vi "SUB-ROM Data convert to table.vi"(4 "ROM Table Ref":refnum<vi>, 5 "ROM Data Ref":refnum<vi>) -> (1 "ROM Table":string[][](table)=[["Device ID", "-", "-"], ["Main Chip", "-", "-"], ["YEAR", "-", "-"], ["Month", "-", "-"], ["Day", "-", "-"], ["Device Type", "-", "-"], ["Manufacturer ID", "-", "-"], ["Cal_Acc. X", "-", "-"], ["Cal_Acc. Y", "-", "-"], ["Cal_Acc. Z", "-", "-"], ["Cal_Gy. X", "-", "-"], ["Cal_Gy. Y", "-", "-"], ["Cal_Gy. Z", "-", "-"], ["Cal_Vol H", "-", "-"], ["Cal_Vol L", "-", "-"], ["Cal_CDC Off 1", "-", "-"], ["Cal_CDC Off 2", "-", "-"], ["Cal_CDC Off 3", "-", "-"], ["Cal_CDC Off 4", "-", "-"], ["Cal_CDC Off 5", "-", "-"], ["Cal_CDC Off 6", "-", "-"], ["Cal_CDC Gain A", "-", "-"], ["Cal_CDC Gain B", "-", "-"]], 2 "ROM Data":T1(array[cluster])=[{"RxOK"=TRUE, "ROM Data"=[255, 255, 255, 255, 255, 255, 255, 255, 255, 255, 255, 255, 255, 255, 255, 255, 2], "Index"=0}, {"RxOK"=TRUE, "ROM Data"=[255, 255, 255, 255, 255, 255, 255, 255, 255, 255, 255, 255, 255, 255, 255, 255, 5], "Index"=1}, {"RxOK"=TRUE, "ROM Data"=[255, 255, 255, 255, 255, 255, 255, 255, 255, 255, 255, 255, 255, 255, 255, 255, 8], "Index"=2}] {"Index" format="%02x"; "ROM Data" format="%02x"})   [LabVIEW 2015]
panel:
  out "Last Index":i32=2
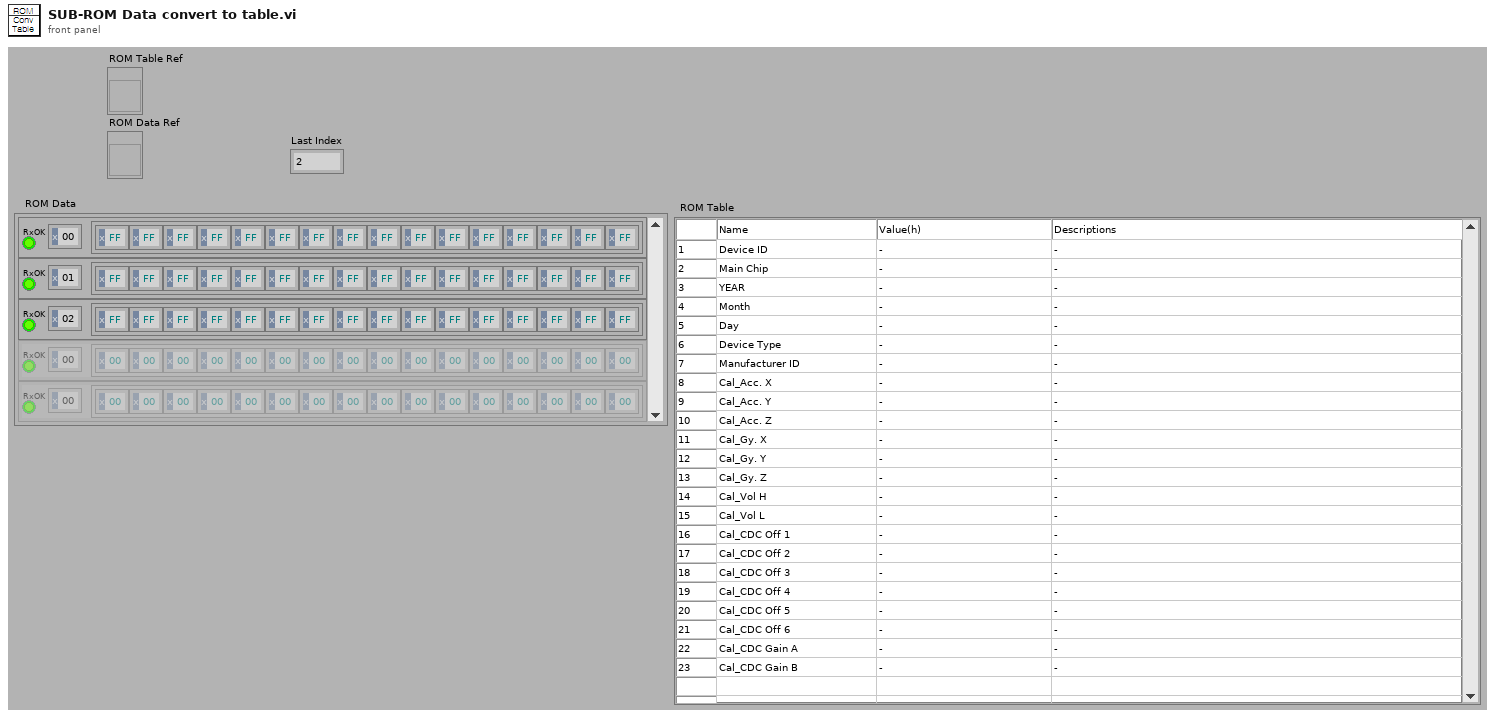
[diagram p1: front panel]
types:
  T1 = cluster{"RxOK":bool, "ROM Data":u8[], "Index":u8}[]
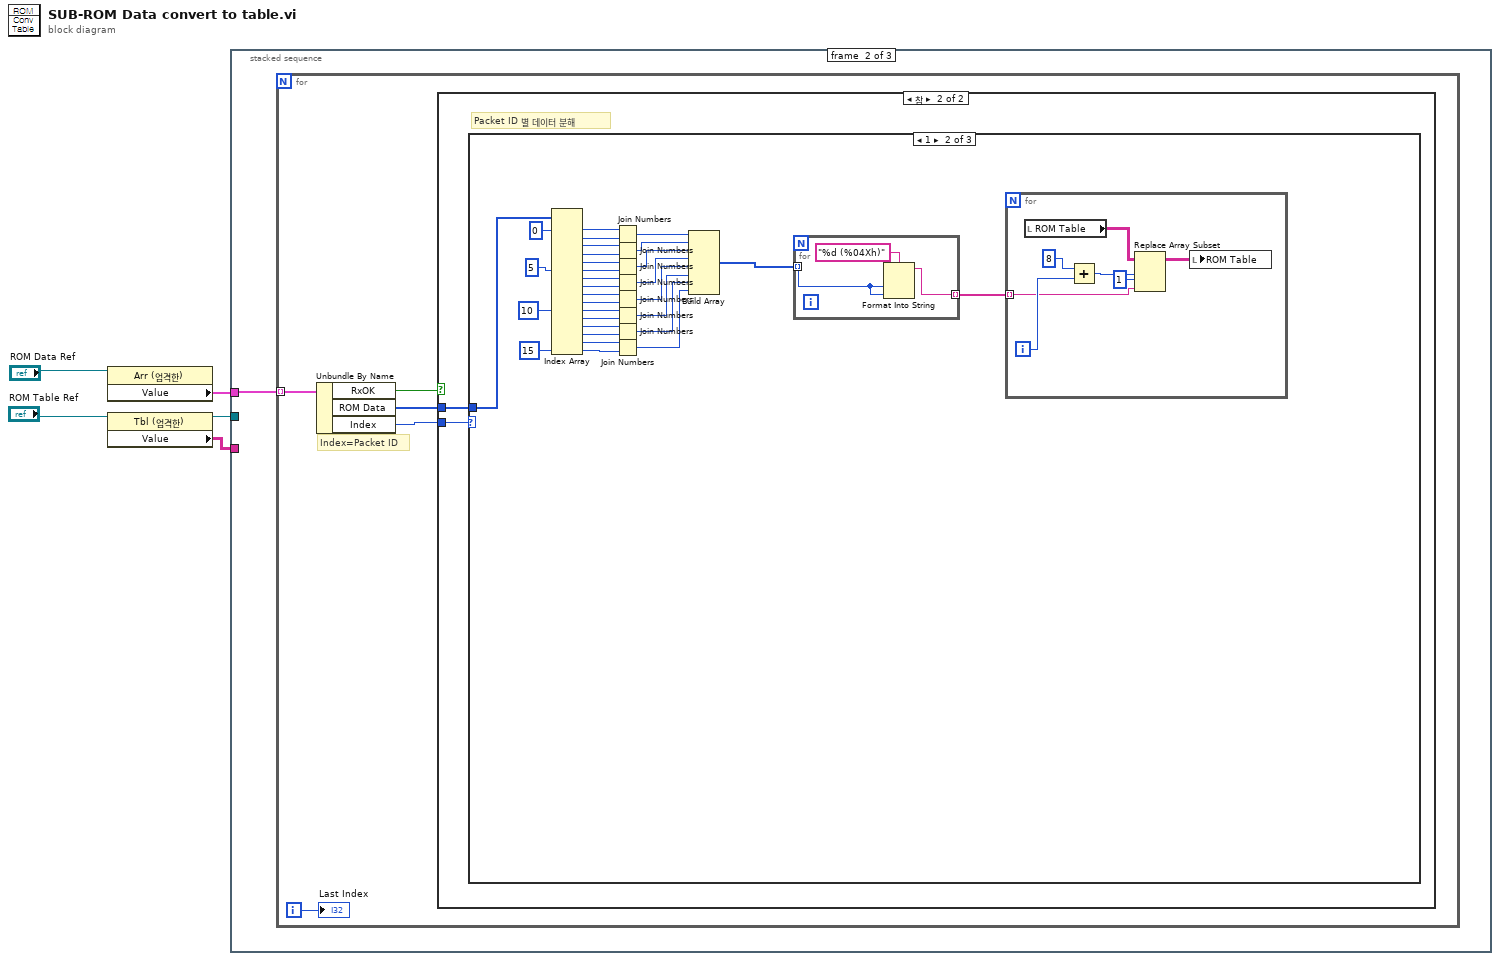
[diagram p0: block diagram]
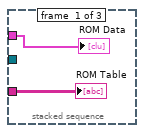
[diagram p2: hidden frame]
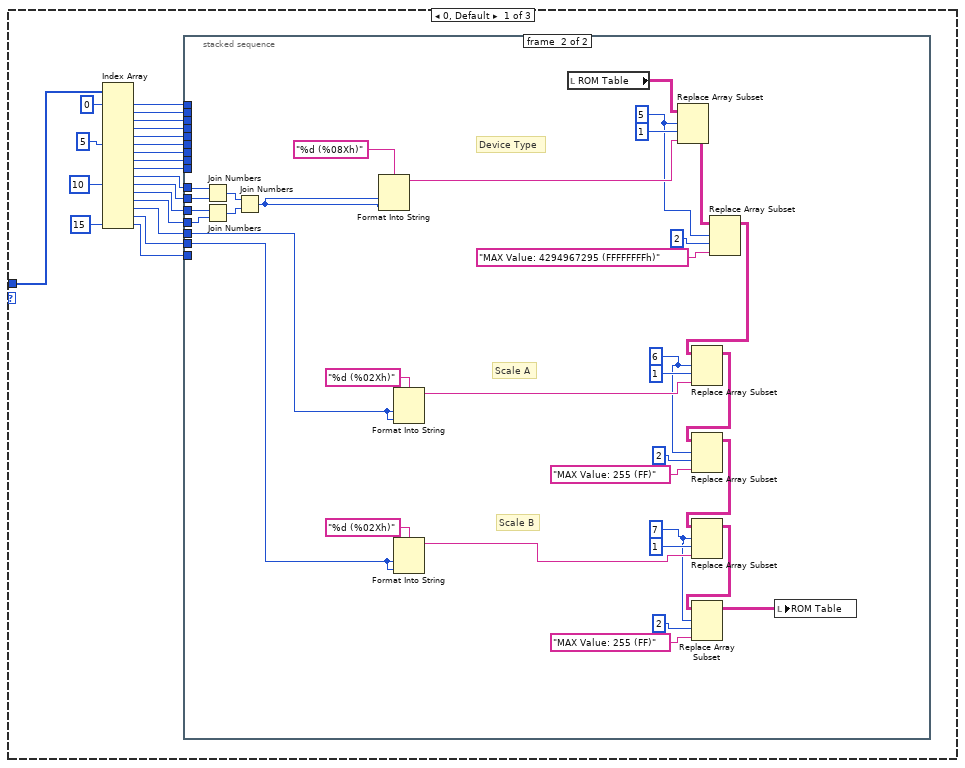
[diagram p4: hidden frame]
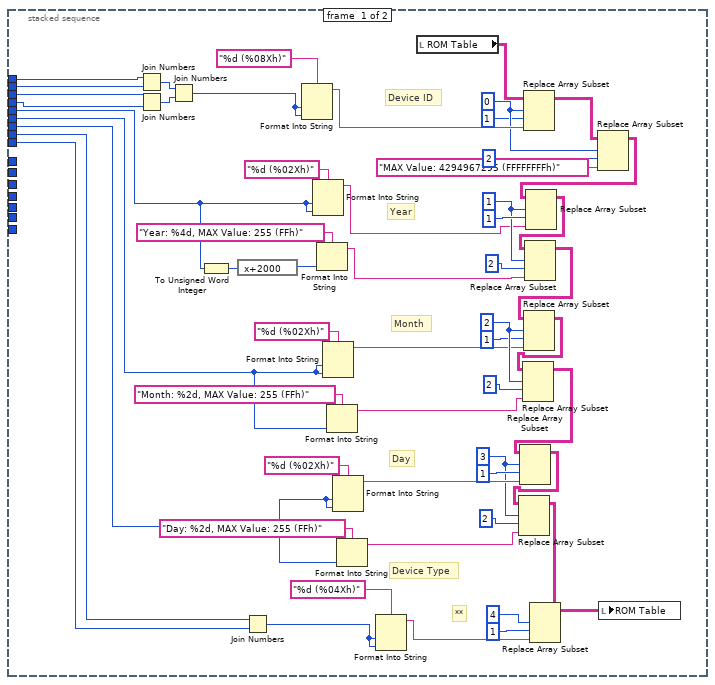
[diagram p5: hidden frame]
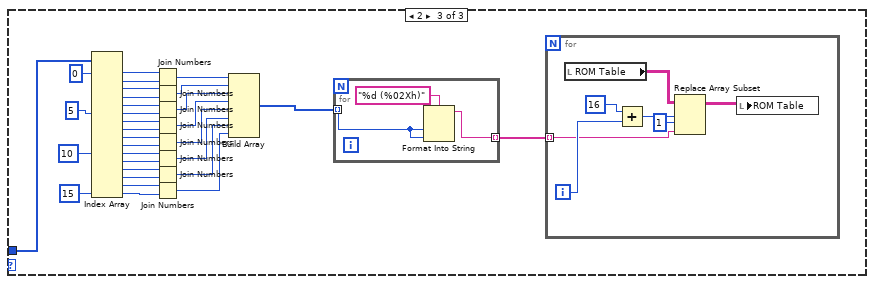
[diagram p6: hidden frame]
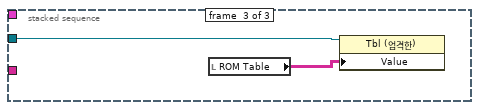
[diagram p7: hidden frame]
diagram:
  n1 = property class="Arr (엄격한)"(reference="ROM Data Ref") -> ("Value"=w3:T1)  [unwired: 1 in, 2 out]
  n2 = property class="Tbl (엄격한)"(reference="ROM Table Ref") -> (reference out=w1:refnum<vi>, "Value"=w2:string[][])  [unwired: 1 in, 1 out]
  n3 = stacked-sequence {
    tunnel: w3 -> [w7 w8 _]
    tunnel: w2 -> [w6 _ _]
    tunnel: w1 -> [_ _ w210]
    frame #0 {
      "ROM Data" <- w7
      "ROM Table" <- w6
    }
    frame #1 {
      n4 = for {
        tunnel: w8 -> [w13] mode=indexing
        i -> [w9]
        # "Index=Packet ID"
        n5 = Unbundle By Name(w13) -> ("RxOK"=w11:bool, "ROM Data"=w10:u8[], "Index"=w12:u8)
        n6 = case shown="참" w11 {
          tunnel: w12 -> [_ w15]
          tunnel: w10 -> [_ w14]
          frame False {
          }
          frame True {
            # "Packet ID 별 데이터 분해"
            n7 = case shown="1" w15 {
              tunnel: w14 -> [w32 w153 w194]
              frame 0, Default {
                n8 = Index Array(array=w32, index #1=0 ("인덱스"), index #6=5 ("인덱스"), index #11=10 ("인덱스"), index #16=15 ("인덱스")) -> (element #1=w31:u8, element #2=w30:u8, element #3=w29:u8, element #4=w28:u8, element #5=w27:u8, element #6=w26:u8, element #7=w25:u8, element #8=w24:u8, element #9=w23:u8, element #10=w22:u8, element #11=w21:u8, element #12=w20:u8, element #13=w19:u8, element #14=w18:u8, element #15=w17:u8, element #16=w16:u8)  [unwired: 12 in]
                n9 = stacked-sequence {
                  tunnel: w31 -> [w87 _]
                  tunnel: w30 -> [w86 _]
                  tunnel: w29 -> [w85 _]
                  tunnel: w28 -> [w84 _]
                  tunnel: w27 -> [w78 _]
                  tunnel: w26 -> [w64 _]
                  tunnel: w25 -> [w52 _]
                  tunnel: w24 -> [w46 _]
                  tunnel: w23 -> [w45 _]
                  tunnel: w22 -> [_ w124]
                  tunnel: w21 -> [_ w123]
                  tunnel: w20 -> [_ w122]
                  tunnel: w19 -> [_ w121]
                  tunnel: w18 -> [_ w113]
                  tunnel: w17 -> [_ w110]
                  tunnel: w16 -> [_ _]
                  frame #0 {
                    w56 = 3 ("인덱스 (행)")
                    w69 = 2 ("인덱스 (행)")
                    w75 = 1 ("인덱스 (행)")
                    w42 = 0 ("인덱스 (행)")
                    # "Device Type"
                    # "**"
                    # "Day"
                    # "Month"
                    # "Year"
                    # "Device ID"
                    n10 = Join Numbers(hi=w87, lo=w86) -> ((hi.lo)=w88:u16)
                    n11 = Join Numbers(hi=w85, lo=w84) -> ((hi.lo)=w89:u16)
                    n12 = Join Numbers(hi=w88, lo=w89) -> ((hi.lo)=w91:u32)
                    n13 = To Unsigned Word Integer(number=w78) -> (unsigned 16bit integer=w79:u16)
                    n14 = expression code="x+2000"(w79) -> (w80:u16)
                    n15 = Join Numbers(hi=w46, lo=w45) -> ((hi.lo)=w50:u16)
                    n16 = Format Into String(format string="%d (%08Xh)" ("포맷 문자열"), w91, w91) -> (resulting string=w83:string)  [unwired: 2 in, 1 out]
                    n17 = Format Into String(format string="%d (%02Xh)" ("포맷 문자열"), w78, w78) -> (resulting string=w73:string)  [unwired: 2 in, 1 out]
                    n18 = Format Into String(format string="Year: %4d, MAX Value: 255 (FFh)" ("포맷 문자열"), w80) -> (resulting string=w72:string)  [unwired: 2 in, 1 out]
                    n19 = Format Into String(format string="%d (%02Xh)" ("포맷 문자열"), w64, w64) -> (resulting string=w67:string)  [unwired: 2 in, 1 out]
                    n20 = Format Into String(format string="Month: %2d, MAX Value: 255 (FFh)" ("포맷 문자열"), w64) -> (resulting string=w71:string)  [unwired: 2 in, 1 out]
                    n21 = Format Into String(format string="%d (%02Xh)" ("포맷 문자열"), w52, w52) -> (resulting string=w59:string)  [unwired: 2 in, 1 out]
                    n22 = Format Into String(format string="Day: %2d, MAX Value: 255 (FFh)" ("포맷 문자열"), w52) -> (resulting string=w54:string)  [unwired: 2 in, 1 out]
                    n23 = Format Into String(format string="%d (%04Xh)" ("포맷 문자열"), w50, w50) -> (resulting string=w48:string)  [unwired: 2 in, 1 out]
                    n24 = local read "ROM Table"() -> (w92:string[][])
                    n25 = Replace Array Subset(array=w92, new element=w83, index (row)=w42, index (col)=1 ("비활성화된 인덱스 (열)")) -> (w44:string[][])
                    n26 = Replace Array Subset(array=w44, new element="MAX Value: 4294967295 (FFFFFFFFh)" ("새 원소/부분배열"), index (row)=w42, index (col)=2 ("비활성화된 인덱스 (열)")) -> (w43:string[][])
                    n27 = Replace Array Subset(array=w43, new element=w73, index (row)=w75, index (col)=1 ("인덱스 (행)")) -> (w74:string[][])
                    n28 = Replace Array Subset(array=w74, new element=w72, index (row)=w75, index (col)=2 ("인덱스 (행)")) -> (w63:string[][])
                    n29 = Replace Array Subset(array=w63, new element=w67, index (row)=w69, index (col)=1 ("인덱스 (행)")) -> (w62:string[][])
                    n30 = Replace Array Subset(array=w62, new element=w71, index (row)=w69, index (col)=2 ("인덱스 (행)")) -> (w53:string[][])
                    n31 = Replace Array Subset(array=w53, new element=w59, index (row)=w56, index (col)=1 ("인덱스 (행)")) -> (w57:string[][])
                    n32 = Replace Array Subset(array=w57, new element=w54, index (row)=w56, index (col)=2 ("인덱스 (행)")) -> (w47:string[][])
                    n33 = Replace Array Subset(array=w47, new element=w48, index (row)=4 ("인덱스 (행)"), index (col)=1 ("인덱스 (행)")) -> (w37:string[][])
                    n34 = local write "ROM Table"(w37) -> ()
                  }
                  frame #1 {
                    w99 = 7 ("인덱스 (행)")
                    w98 = 6 ("인덱스 (행)")
                    w93 = 5 ("인덱스 (행)")
                    # "Scale B"
                    # "Scale A"
                    # "Device Type"
                    n35 = Join Numbers(hi=w124, lo=w123) -> ((hi.lo)=w125:u16)
                    n36 = Join Numbers(hi=w122, lo=w121) -> ((hi.lo)=w126:u16)
                    n37 = Join Numbers(hi=w125, lo=w126) -> ((hi.lo)=w119:u32)
                    n38 = Format Into String(format string="%d (%08Xh)" ("포맷 문자열"), w119, w119) -> (resulting string=w116:string)  [unwired: 2 in, 1 out]
                    n39 = Format Into String(format string="%d (%02Xh)" ("포맷 문자열"), w113, w113) -> (resulting string=w112:string)  [unwired: 2 in, 1 out]
                    n40 = Format Into String(format string="%d (%02Xh)" ("포맷 문자열"), w110, w110) -> (resulting string=w108:string)  [unwired: 2 in, 1 out]
                    n41 = local read "ROM Table"() -> (w117:string[][])
                    n42 = Replace Array Subset(array=w117, new element=w116, index (row)=w93, index (col)=1 ("비활성화된 인덱스 (열)")) -> (w95:string[][])
                    n43 = Replace Array Subset(array=w95, new element="MAX Value: 4294967295 (FFFFFFFFh)" ("새 원소/부분배열"), index (row)=w93, index (col)=2 ("인덱스 (행)")) -> (w94:string[][])
                    n44 = Replace Array Subset(array=w94, new element=w112, index (row)=w98, index (col)=1 ("비활성화된 인덱스 (열)")) -> (w105:string[][])
                    n45 = Replace Array Subset(array=w105, new element="MAX Value: 255 (FF)" ("새 원소/부분배열"), index (row)=w98, index (col)=2 ("인덱스 (행)")) -> (w102:string[][])
                    n46 = Replace Array Subset(array=w102, new element=w108, index (row)=w99, index (col)=1 ("비활성화된 인덱스 (열)")) -> (w101:string[][])
                    n47 = Replace Array Subset(array=w101, new element="MAX Value: 255 (FF)" ("새 원소/부분배열"), index (row)=w99, index (col)=2 ("인덱스 (행)")) -> (w100:string[][])
                    n48 = local write "ROM Table"(w100) -> ()
                  }
                }
              }
              frame 1 {
                n49 = Index Array(array=w153, index #1=0 ("인덱스"), index #6=5 ("인덱스"), index #11=10 ("인덱스"), index #16=15 ("인덱스")) -> (element #1=w152:u8, element #2=w151:u8, element #3=w150:u8, element #4=w149:u8, element #5=w148:u8, element #6=w147:u8, element #7=w146:u8, element #8=w145:u8, element #9=w144:u8, element #10=w143:u8, element #11=w142:u8, element #12=w141:u8, element #13=w140:u8, element #14=w139:u8, element #15=w138:u8, element #16=w137:u8)  [unwired: 12 in]
                n50 = Join Numbers(hi=w152, lo=w151) -> ((hi.lo)=w136:u16)
                n51 = Join Numbers(hi=w150, lo=w149) -> ((hi.lo)=w135:u16)
                n52 = Join Numbers(hi=w148, lo=w147) -> ((hi.lo)=w134:u16)
                n53 = Join Numbers(hi=w146, lo=w145) -> ((hi.lo)=w133:u16)
                n54 = Join Numbers(hi=w144, lo=w143) -> ((hi.lo)=w132:u16)
                n55 = Join Numbers(hi=w142, lo=w141) -> ((hi.lo)=w131:u16)
                n56 = Join Numbers(hi=w140, lo=w139) -> ((hi.lo)=w130:u16)
                n57 = Join Numbers(hi=w138, lo=w137) -> ((hi.lo)=w129:u16)
                n58 = Build Array(w136, w135, w134, w133, w132, w131, w130, w129) -> (w128:u16[])
                n59 = for {
                  tunnel: w128 -> [w166] mode=indexing
                  tunnel: [w165] -> w127 mode=indexing
                  n60 = Format Into String(format string="%d (%04Xh)" ("포맷 문자열"), w166, w166) -> (resulting string=w165:string)  [unwired: 2 in, 1 out]
                }
                n61 = for {
                  tunnel: w127 -> [w161] mode=indexing
                  i -> [w162]
                  n62 = local read "ROM Table"() -> (w164:string[][])
                  n63 = Add(x=8, y=w162) -> (x+y=w159:i32)
                  n64 = Replace Array Subset(array=w164, new element=w161, index (row)=w159, index (col)=1 ("비활성화된 인덱스 (열)")) -> (w158:string[][])
                  n65 = local write "ROM Table"(w158) -> ()
                }
              }
              frame 2 {
                n66 = Index Array(array=w194, index #1=0 ("인덱스"), index #6=5 ("인덱스"), index #11=10 ("인덱스"), index #16=15 ("인덱스")) -> (element #1=w193:u8, element #2=w192:u8, element #3=w191:u8, element #4=w190:u8, element #5=w189:u8, element #6=w188:u8, element #7=w187:u8, element #8=w186:u8, element #9=w185:u8, element #10=w184:u8, element #11=w183:u8, element #12=w182:u8, element #13=w181:u8, element #14=w180:u8, element #15=w179:u8, element #16=w178:u8)  [unwired: 12 in]
                n67 = Join Numbers(hi=w193, lo=w192) -> ((hi.lo)=w177:u16)
                n68 = Join Numbers(hi=w191, lo=w190) -> ((hi.lo)=w176:u16)
                n69 = Join Numbers(hi=w189, lo=w188) -> ((hi.lo)=w175:u16)
                n70 = Join Numbers(hi=w187, lo=w186) -> ((hi.lo)=w174:u16)
                n71 = Join Numbers(hi=w185, lo=w184) -> ((hi.lo)=w173:u16)
                n72 = Join Numbers(hi=w183, lo=w182) -> ((hi.lo)=w172:u16)
                n73 = Join Numbers(hi=w181, lo=w180) -> ((hi.lo)=w171:u16)
                n74 = Join Numbers(hi=w179, lo=w178) -> ((hi.lo)=w170:u16)
                n75 = Build Array(w177, w176, w175, w174, w173, w172, w171, w170) -> (w169:u16[])
                n76 = for {
                  tunnel: w169 -> [w207] mode=indexing
                  tunnel: [w206] -> w168 mode=indexing
                  n77 = Format Into String(format string="%d (%02Xh)" ("포맷 문자열"), w207, w207) -> (resulting string=w206:string)  [unwired: 2 in, 1 out]
                }
                n78 = for {
                  tunnel: w168 -> [w202] mode=indexing
                  i -> [w203]
                  n79 = local read "ROM Table"() -> (w205:string[][])
                  n80 = Add(x=16, y=w203) -> (x+y=w200:i32)
                  n81 = Replace Array Subset(array=w205, new element=w202, index (row)=w200, index (col)=1 ("비활성화된 인덱스 (열)")) -> (w199:string[][])
                  n82 = local write "ROM Table"(w199) -> ()
                }
              }
            }
          }
        }
        "Last Index" <- w9
      }
    }
    frame #2 {
      n83 = local read "ROM Table"() -> (w209:string[][])
      n84 = property class="Tbl (엄격한)"(reference=w210, "Value"=w209) -> ()  [unwired: 1 in, 2 out]
    }
  }
